vi "Actual Sample Rate.vi"(8 "error in (no error)":errorcluster, 11 "CS++Scope":refnum<class "CS++Scope.lvclass">) -> (0 "error out":errorcluster, 2 "sample rate":dbl[unit] caption="sample rate (samples/s)" format="%^.2e", 3 "CS++Scope out":refnum<class "CS++Scope.lvclass">)   [LabVIEW 2014, in "CS++Scope.lvlib" / "CS++Scope.lvclass"]
doc: "This VI returns the effective sample rate of the acquired waveform using the current configuration in samples per second."
uses:
  CS++Scope.lvclass
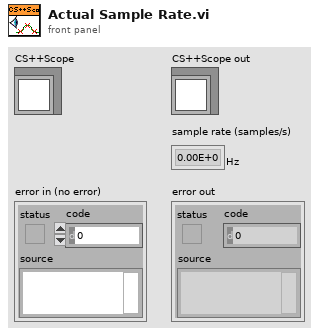
[diagram p1: front panel]
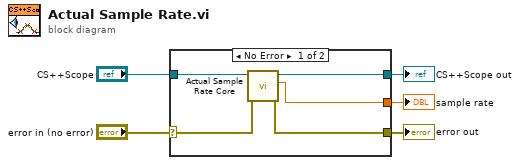
[diagram p0: block diagram]
diagram:
  n1 = case shown="No Error" "error in (no error)" {
    selector: "error in (no error)" -> [w8 w12]
    tunnel: [w7 w12] -> w4
    tunnel: [w9 w11] -> w3
    tunnel: "CS++Scope" -> [w10 w11]
    tunnel: [w6 _] -> w1
    frame No Error {
      n2 = call-dynamic "Actual Sample Rate Core.vi"("error in (no error)"=w8, "CS++Scope"=w10) -> ("error out"=w7:errorcluster, "sample rate"=w6:dbl[unit], "CS++Scope out"=w9:refnum<class "CS++Scope.lvclass">)  [unwired: 7 in]
    }
    frame Error {
    }
  }
  "error out" <- w4
  "sample rate" <- w1
  "CS++Scope out" <- w3
